vi "fpga_Channel Switch.vi"(0 "lower Limits":fxp<+/-,24,1>[](array[numeric])=[0.9999998807907104, 0.9999998807907104, 0.9999998807907104, 0.5, 0.5, 0.5, 0.0], 1 "signals in":fxp<+/-,24,1>[](array[numeric])=[0.0, 0.0, 0.0, 0.0, 0.0, 0.0, 0.0], 2 "window length (10000)":u16=10000, 5 "upper Limits":fxp<+/-,24,1>[](array[numeric])=[0.9999998807907104, 0.9999998807907104, 0.9999998807907104, 0.9999998807907104, 0.9999998807907104, 0.9999998807907104, 0.0], 9 "channel index":i32=-1, 11 "max index":u32=2, 12 "previous channel index":i32=-1) -> (6 "resampling channel index":i32)   [LabVIEW 2014]
uses:
  <vilib>/rvi/FXPMathLib/basic elements/FxpAddSub/XNode/nifxpmath_AddSub.xnode
  <vilib>/rvi/FXPMathLib/sim/FxpSim.dll
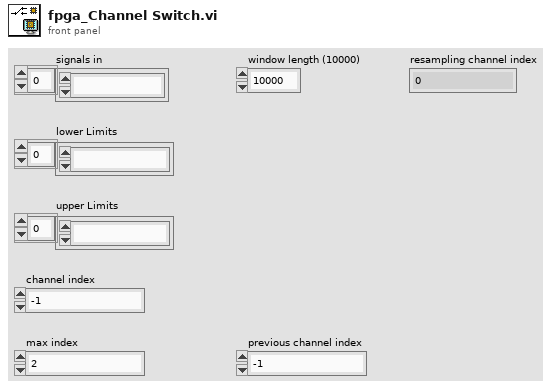
[diagram p1: front panel]
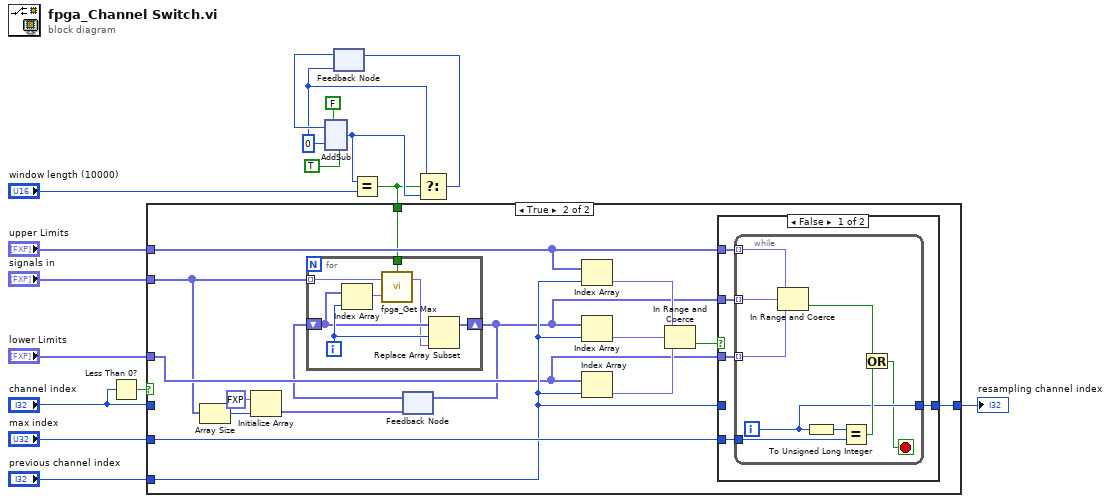
[diagram p0: block diagram]
diagram:
  w6 = u16 0 ("y")
  n1 = Less Than 0?(x="channel index") -> (x < 0?=w10:bool)
  n2 = feedback #1(w6) -> (w8:u16)
  n3 = xnode "AddSub"("x"=w8, "y"=w6, "carry-in"=TRUE, "use zero instead of x"=FALSE) -> ("s"=w5:u16)  [unwired: 1 out]
  n4 = Equal?(x=w5, y="window length (10000)") -> (x = y?=w2:bool)
  n5 = case shown="True" w10 {
    tunnel: [w17 w33] -> w16
    tunnel: "max index" -> [_ w32]
    tunnel: "channel index" -> [w17 _]
    tunnel: "upper Limits" -> [_ w26]
    tunnel: "lower Limits" -> [_ w24]
    tunnel: "signals in" -> [_ w23]
    tunnel: "previous channel index" -> [_ w27]
    tunnel: w2 -> [_ w25]
    frame False {
    }
    frame True {
      n6 = Array Size(array=w23) -> (size(s)=w21:i32)
      n7 = Initialize Array(fxp<+/-,24,1> 0.0 ("fixed-point type"), w21) -> (w20:fxp<+/-,24,1>[])
      n8 = feedback #2(w20) -> (w19:fxp<+/-,24,1>[])
      n9 = for {
        tunnel: w25 -> [w40]
        tunnel: w23 -> [w39] mode=indexing
        shift-right: [w37] -> w18
        shift-left: w19 -> [w35]
        i -> [w36]
        n10 = Index Array(array=w35, index=w36) -> (element=w38:fxp<+/-,24,1>)
        n11 = call <vilib>:"fpga_Get Max.vi"("previous max value"=w38, "signal in"=w39, "reset? (F)"=w40) -> ("current max value"=w34:fxp<+/-,24,1>)  [unwired: 1 in]
        n12 = Replace Array Subset(array=w35, new element=w34, index=w36) -> (w37:fxp<+/-,24,1>[])
      }
      n13 = feedback-in #2(w18) -> ()
      n14 = Index Array(array=w26, index=w27) -> (element=w31:fxp<+/-,24,1>)
      n15 = Index Array(array=w18, index=w27) -> (element=w29:fxp<+/-,24,1>)
      n16 = Index Array(array=w24, index=w27) -> (element=w30:fxp<+/-,24,1>)
      n17 = In Range and Coerce(upper limit=w31, x=w29, lower limit=w30) -> (In Range?=w28:bool)  [unwired: 1 out]
      n18 = case shown="False" w28 {
        tunnel: w32 -> [w45 _]
        tunnel: w27 -> [_ w55]
        tunnel: [w44 w55] -> w33
        tunnel: w26 -> [w43 _]
        tunnel: w24 -> [w42 _]
        tunnel: w18 -> [w41 _]
        frame False {
          n19 = while {
            tunnel: w45 -> [w54]
            tunnel: [w47] -> w44
            tunnel: w43 -> [w50] mode=indexing
            tunnel: w42 -> [w49] mode=indexing
            tunnel: w41 -> [w51] mode=indexing
            i -> [w47]
            stop <- w46 stop-if-true
            n20 = In Range and Coerce(upper limit=w50, x=w51, lower limit=w49) -> (In Range?=w48:bool)  [unwired: 1 out]
            n21 = To Unsigned Long Integer(number=w47) -> (unsigned 32bit integer=w52:u32)
            n22 = Equal?(x=w52, y=w54) -> (x = y?=w53:bool)
            n23 = Or(x=w48, y=w53) -> (x .or. y?=w46:bool)
          }
        }
        frame True {
        }
      }
    }
  }
  "resampling channel index" <- w16
  n24 = Select(t=w6, s=w2, f=w5) -> (s? t:f=w4:u16)
  n25 = feedback-in #1(w4) -> ()
